vi "Get Angle Distance.vi"(8 "Target":dbl, 11 "Current":dbl) -> (1 "Distance":dbl)   [LabVIEW 2016]
panel:
  out "Current Angle":dbl(knob) scale=-180.0..180.0
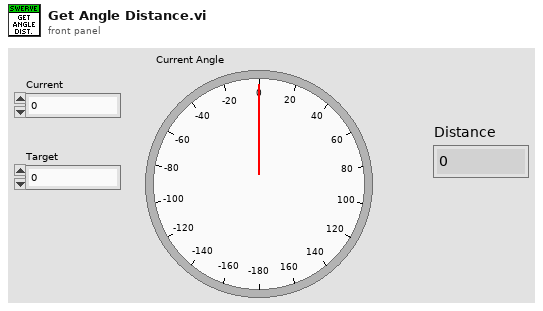
[diagram p1: front panel]
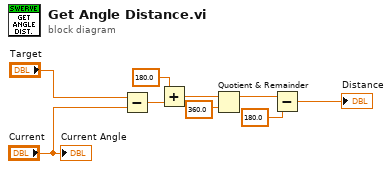
[diagram p0: block diagram]
diagram:
  n1 = Subtract(x="Target", y="Current") -> (x-y=w7:dbl)
  n2 = Add(x=180.0, y=w7) -> (x+y=w5:dbl)
  n3 = Quotient & Remainder(x=w5, y=360.0) -> (x-y*floor(x/y)=w3:dbl)  [unwired: 1 out]
  n4 = Subtract(x=w3, y=180.0) -> (x-y=→"Distance":dbl)
  "Current Angle" <- "Current"
